vi "Preview.vi"(8 "error in (no error)":errorcluster, 10 "Project":refnum<vi>, 11 "IB_Tree_Item_Proj_Build in":refnum<class "IB_Tree_Item_Proj_Build.lvclass">) -> (0 "error out":errorcluster, 2 "first preview?":bool, 3 "IB_Tree_Item_Proj_Build out":refnum<class "IB_Tree_Item_Proj_Build.lvclass">)   [LabVIEW 2020, in "IB_Tree_Item_Proj_Build.lvclass"]
uses:
  <vilib>/AppBuilder/IB_Classes/Tree_Item_Proj_Build/IB_Tree_Item_Proj_Build.lvclass
  <vilib>/AppBuilder/IB_Classes/Tree_Item_Proj_Build/IB_Tree_Item_Proj_Build.lvclass/IB_Tree_Item_Proj_Build.ctl
  <vilib>/AppBuilder/IB_Classes/Tree_Item_Proj/IB_Tree_Item_Proj.lvclass
  <vilib>/AppBuilder/IB_Classes/Tree_Item_Proj_Container/IB_Tree_Item_Proj_Container.lvclass
  <vilib>/AppBuilder/IB_Classes/Tree_Item_Proj_Contained_File/IB_Tree_Item_Proj_Contained_File.lvclass
  <vilib>/AppBuilder/IB_Classes/Tree_Item_Virtual_Folder/IB_Tree_Item_Virtual_Folder.lvclass
  <vilib>/AppBuilder/IB_Classes/Tree_Item/IB_Tree_Item.lvclass
  e:/builds/penguin/labview/branches/2020/dev/dist/vi.lib/AppBuilder/IB_Classes/Tree_Item_Proj_Container/IB_Tree_Item_Proj_Container.lvclass
  e:/builds/penguin/labview/branches/2020/dev/dist/vi.lib/AppBuilder/IB_Classes/Tree_Item_Proj/IB_Tree_Item_Proj.lvclass
  e:/builds/penguin/labview/branches/2020/dev/dist/vi.lib/AppBuilder/IB_Classes/Tree_Item/IB_Tree_Item.lvclass
  e:/builds/penguin/labview/branches/2020/dev/dist/vi.lib/AppBuilder/IB_Classes/Tree_Item_Proj_Build/IB_Tree_Item_Proj_Build.lvclass
  e:/builds/penguin/labview/branches/2020/dev/dist/vi.lib/AppBuilder/IB_Classes/Tree_Item_Proj_File/IB_Tree_Item_Proj_File.lvclass
  e:/builds/penguin/labview/branches/2020/dev/dist/vi.lib/AppBuilder/IB_Classes/Tree_Item_Proj_Contained_File/IB_Tree_Item_Proj_Contained_File.lvclass
  e:/builds/penguin/labview/branches/2020/dev/dist/vi.lib/AppBuilder/IB_Classes/Tree_Item_Virtual_Folder/IB_Tree_Item_Virtual_Folder.lvclass
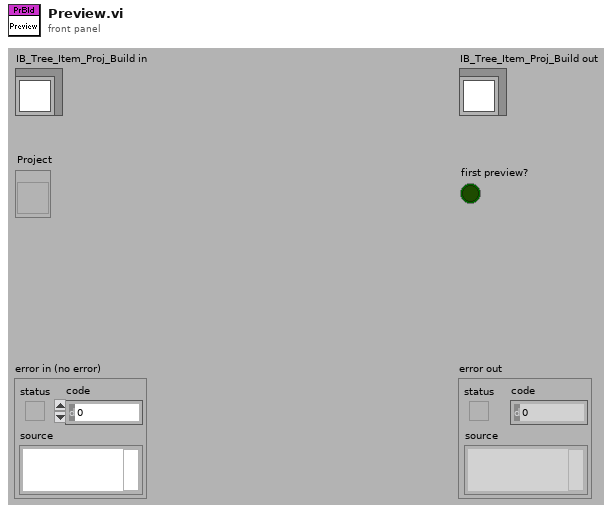
[diagram p1: front panel]
types:
  T1 = typedef "IB_Tree_Item_Proj.ctl" = cluster{"itemID":string, "path":path}
  T2 = typedef "SRdB_Bld.ctl" = cluster{"ItemID":string, "FileItemIDs":string[], "RelPaths":string[], "AbsPaths":path[], "preview error?":bool, "Dependencies":T3[]}
  T3 = typedef "AB_Dependency.ctl" = cluster{"path":path, "delimited name":string, "type":T4}
  T4 = typedef "NI_FileType.lvlib/LVFileType.ctl" = enum32{"Invalid file", "Unknown type", "Instrument", "Control", "Polymorphic VI", "Project", "Library", "LVClass", "XControl", "XNode", "Shared library", ".NET assembly", "ActiveX interface", "CIN", "Run-time menu", "Palette menu", "Help file", "LLB", "XNode Edit Dependency", "Class Private Data Control", "Statechart", "MathScript .m file", "Ladder Diagram", "LVLibp", "XNode Build Dependency"}
  T5 = typedef "IB_Tree_Item.ctl" = cluster{"symbol index":i32, "child tag":string, "parentTag":string, "left cell name":string}
  T6 = typedef "IB_Tree_Item_Proj_Contained_File.ctl" = cluster{"virt folders":refnum<class "IB_Tree_Item_Virtual_Folder.lvclass">[]}
  T7 = typedef "IB_Tree_Item_Proj_Container.ctl" = cluster{"ctr files":refnum<class "IB_Tree_Item_Proj_Contained_File.lvclass">[], "previewed?":bool, "expanded?":bool, "preview error?":bool}
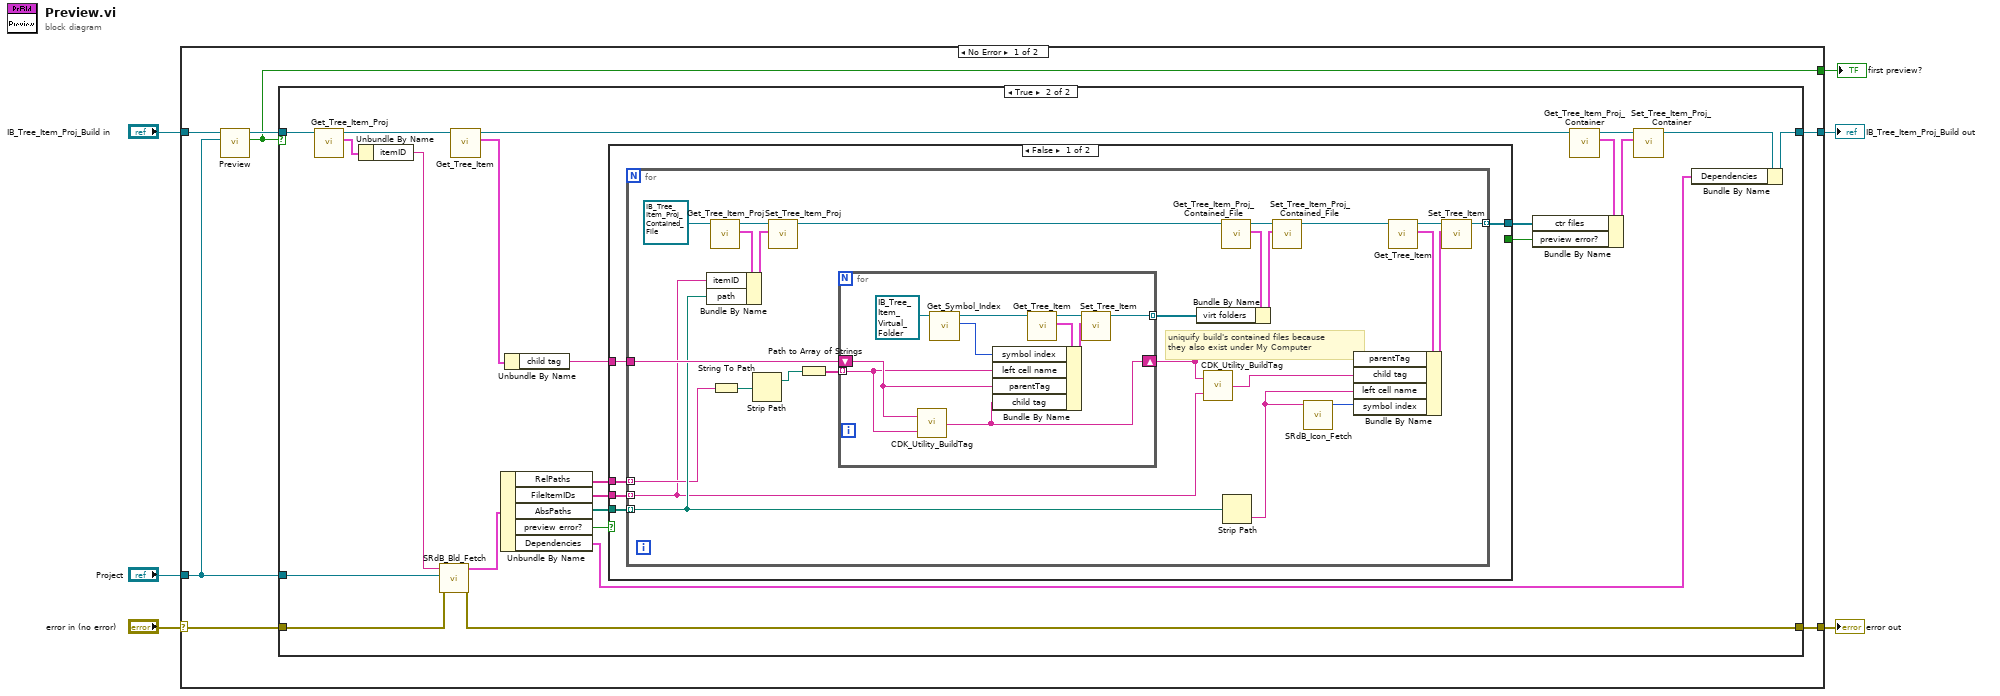
[diagram p0: block diagram]
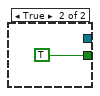
[diagram p3: hidden frame]
diagram:
  n1 = case shown="No Error" "error in (no error)" {
    selector: "error in (no error)" -> [w12 w81]
    tunnel: [w11 w81] -> w5
    tunnel: [w13 w80] -> w3
    tunnel: "IB_Tree_Item_Proj_Build in" -> [w10 w80]
    tunnel: "Project" -> [w8 _]
    tunnel: [w7 _] -> w1
    frame No Error {
      n2 = call-parent "Preview.vi"("Project"=w8, "IB_Tree_Item_Proj_Container in"=w10) -> ("first preview?"=w7:bool, "IB_Tree_Item_Proj_Container out"=w9:refnum<class "IB_Tree_Item_Proj_Build.lvclass">)  [unwired: 1 in, 7 out]
      n3 = case shown="True" w7 {
        tunnel: [w14 w16] -> w13
        tunnel: w12 -> [w15 w38]
        tunnel: [w15 w37] -> w11
        tunnel: w9 -> [w14 w22]
        tunnel: w8 -> [_ w21]
        frame False {
        }
        frame True {
          n4 = call <vilib>:"Get_Tree_Item_Proj.vi"("IB_TreeProjectItem in"=w22) -> ("data"=w36:T1, "IB_TreeProjectItem out"=w27:refnum<class "IB_Tree_Item_Proj_Build.lvclass">)  [unwired: 1 in, 8 out]
          n5 = Unbundle By Name(w36) -> ("itemID"=w31:string)
          n6 = call <resource>:"SRdB_Bld_Fetch.vi"("error in (no error)"=w38, "Project"=w21, "itemID"=w31) -> ("error out"=w37:errorcluster, "build"=w30:T2)  [unwired: 1 in, 6 out]
          n7 = call <vilib>:"Get_Tree_Item.vi"("IB_TreeItem in"=w27) -> ("data"=w25:T5, "IB_TreeItem out"=w26:refnum<class "IB_Tree_Item_Proj_Build.lvclass">)  [unwired: 1 in, 8 out]
          n8 = Unbundle By Name(w30) -> ("RelPaths"=w23:string[], "FileItemIDs"=w28:string[], "AbsPaths"=w29:path[], "preview error?"=w20:bool, "Dependencies"=w18:T3[])
          n9 = Unbundle By Name(w25) -> ("child tag"=w24:string)
          n10 = case shown="False" w20 {
            tunnel: [w43 _] -> w32
            tunnel: w29 -> [w42 _]
            tunnel: w28 -> [w41 _]
            tunnel: w24 -> [w40 _]
            tunnel: w23 -> [w39 _]
            tunnel: [_ TRUE] -> w19
            frame False {
              n11 = for {
                tunnel: [w55] -> w43 mode=indexing
                tunnel: w42 -> [w53] mode=indexing
                tunnel: w41 -> [w45] mode=indexing
                tunnel: w40 -> [w54]
                tunnel: w39 -> [w50] mode=indexing
                # "uniquify build's contained files because\nthey also exist under My Computer"
                n12 = call <vilib>:"Get_Tree_Item_Proj.vi"("IB_TreeProjectItem in"=refnum<class "IB_Tree_Item_Proj_Contained_File.lvclass"> refnum ("IB_Tree_Item_Proj_Contained_File.lvclass")) -> ("data"=w60:T1, "IB_TreeProjectItem out"=w59:refnum<class "IB_Tree_Item_Proj_Contained_File.lvclass">)  [unwired: 1 in, 8 out]
                n13 = Bundle By Name(cluster=w60, "itemID"=w45, "path"=w53) -> (w58:T1)
                n14 = String To Path(string=w50) -> (path=w49:path)
                n15 = Strip Path(path=w49) -> (stripped path=w48:path)  [unwired: 1 out]
                n16 = call <vilib>:"Set_Tree_Item_Proj.vi"("data"=w58, "IB_TreeProjectItem in"=w59) -> ("IB_TreeProjectItem out"=w63:refnum<class "IB_Tree_Item_Proj_Contained_File.lvclass">)  [unwired: 1 in, 8 out]
                n17 = Path to Array of Strings(0:w48) -> (2:w47:string[])  [unwired: 1 out]
                n18 = for {
                  tunnel: [w78] -> w65 mode=indexing
                  tunnel: w47 -> [w75] mode=indexing
                  shift-right: [w77] -> w46
                  shift-left: w54 -> [w76]
                  n19 = call <resource>:"CDK_Utility_BuildTag.vi"("name or relative path"=w75, "BasePath"=w76) -> ("appended path"=w77:string)
                  n20 = call-dynamic "Get_Symbol_Index.vi"("IB_TreeVirtFolderItem in"=refnum<class "IB_Tree_Item_Virtual_Folder.lvclass"> refnum ("IB_Tree_Item_Virtual_Folder.lvclass")) -> ("symbol index"=w69:i32, "IB_TreeVirtFolderItem out"=w70:refnum<class "IB_Tree_Item_Virtual_Folder.lvclass">)  [unwired: 1 in, 8 out]
                  n21 = call <vilib>:"Get_Tree_Item.vi"("IB_TreeItem in"=w70) -> ("data"=w73:T5, "IB_TreeItem out"=w74:refnum<class "IB_Tree_Item_Virtual_Folder.lvclass">)  [unwired: 1 in, 8 out]
                  n22 = Bundle By Name(cluster=w73, "symbol index"=w69, "left cell name"=w75, "parentTag"=w76, "child tag"=w77) -> (w72:T5)
                  n23 = call <vilib>:"Set_Tree_Item.vi"("data"=w72, "IB_TreeItem in"=w74) -> ("IB_TreeItem out"=w78:refnum<class "IB_Tree_Item_Virtual_Folder.lvclass">)  [unwired: 1 in, 8 out]
                }
                n24 = call <resource>:"CDK_Utility_BuildTag.vi"("name or relative path"=w45, "BasePath"=w46) -> ("appended path"=w44:string)
                n25 = call <vilib>:"Get_Tree_Item_Proj_Contained_File.vi"("IB_Tree_Item_Proj_Contained_File in"=w63) -> ("data"=w67:T6, "IB_Tree_Item_Proj_Contained_File out"=w68:refnum<class "IB_Tree_Item_Proj_Contained_File.lvclass">)  [unwired: 1 in, 8 out]
                n26 = Bundle By Name(cluster=w67, "virt folders"=w65) -> (w66:T6)
                n27 = Strip Path(path=w53) -> (name=w52:string)  [unwired: 1 out]
                n28 = call <vilib>:"Set_Tree_Item_Proj_Contained_File.vi"("data"=w66, "IB_Tree_Item_Proj_Contained_File in"=w68) -> ("IB_Tree_Item_Proj_Contained_File out"=w56:refnum<class "IB_Tree_Item_Proj_Contained_File.lvclass">)  [unwired: 1 in, 8 out]
                n29 = call <resource>:"SRdB_Icon_Fetch.vi"("filename"=w52) -> ("symbol index"=w51:i32)  [unwired: 1 in, 9 out]
                n30 = call <vilib>:"Get_Tree_Item.vi"("IB_TreeItem in"=w56) -> ("data"=w62:T5, "IB_TreeItem out"=w64:refnum<class "IB_Tree_Item_Proj_Contained_File.lvclass">)  [unwired: 1 in, 8 out]
                n31 = Bundle By Name(cluster=w62, "parentTag"=w46, "child tag"=w44, "left cell name"=w52, "symbol index"=w51) -> (w61:T5)
                n32 = call <vilib>:"Set_Tree_Item.vi"("data"=w61, "IB_TreeItem in"=w64) -> ("IB_TreeItem out"=w55:refnum<class "IB_Tree_Item_Proj_Contained_File.lvclass">)  [unwired: 1 in, 8 out]
              }
            }
            frame True {
            }
          }
          n33 = call <vilib>:"Get_Tree_Item_Proj_Container.vi"("IB_Tree_Item_Proj_Container in"=w26) -> ("data"=w34:T7, "IB_Tree_Item_Proj_Container out"=w35:refnum<class "IB_Tree_Item_Proj_Build.lvclass">)  [unwired: 1 in, 8 out]
          n34 = Bundle By Name(cluster=w34, "ctr files"=w32, "preview error?"=w19) -> (w33:T7)
          n35 = call <vilib>:"Set_Tree_Item_Proj_Container.vi"("data"=w33, "IB_Tree_Item_Proj_Container in"=w35) -> ("IB_Tree_Item_Proj_Container out"=w17:refnum<class "IB_Tree_Item_Proj_Build.lvclass">)  [unwired: 1 in, 8 out]
          n36 = Bundle By Name(cluster=w17, "Dependencies"=w18) -> (w16:refnum<class "IB_Tree_Item_Proj_Build.lvclass">)
        }
      }
    }
    frame Error {
    }
  }
  "error out" <- w5
  "IB_Tree_Item_Proj_Build out" <- w3
  "first preview?" <- w1
